vi "Parse Results (table).vi"(8 "error in (no error)":errorcluster, 11 "Instrument.Lockin":refnum<class "Instrument.Lockin.lvclass">) -> (0 "error out":errorcluster, 1 "Table":string[][](table), 2 "Results (Dictionary)":cluster{"key":string, "value":dbl}[](array[cluster]), 3 "Instrument.Lockin out":refnum<class "Instrument.Lockin.lvclass">)   [LabVIEW 2019, in "Instrument.Lockin.lvclass"]
uses:
  Instrument.Lockin.lvclass
  Typedefs/Results Type--Enum.ctl
  Instrument.Lockin.lvclass/Instrument.Lockin.ctl
  Instrument.DAQ/Typedefs/DAQ.Config.AI.Range--enum.ctl
  Instrument.DAQ/Instrument.DAQ.lvclass
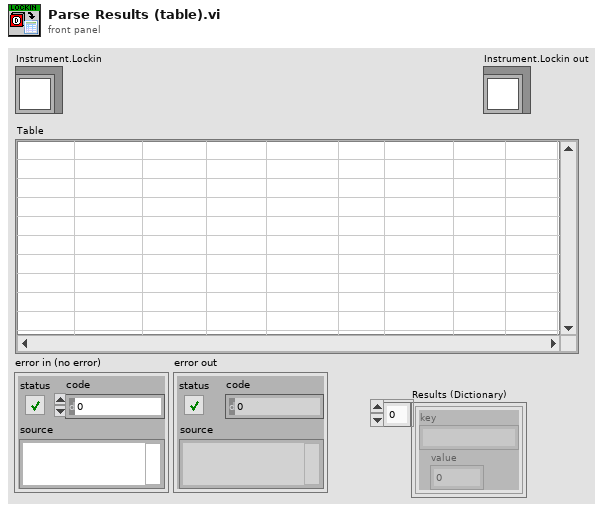
[diagram p1: front panel]
types:
  T1 = typedef "Instrument.Lockin.lvclass/Results Type--Enum.ctl" = enum16{"X", "Y", "R", "Theta", "Mean"}
  T2 = enum32{"Bad", "Idle", "Run top level", "Running"}
  T3 = typedef "Instrument.DAQ.lvclass/DAQ.Config.AI--Cluster--Array.ctl" = T4[]
  T4 = typedef "Instrument.DAQ.lvclass/DAQ.Config.AI--Cluster.ctl" = cluster{"Channels":tag, "Coupling":T5, "Range":T6, "input terminal configuration":i32, "Type":T7}
  T5 = typedef "Instrument.DAQ.lvclass/DAQ.Config.AI.Coupling--enum.ctl" = u16
  T6 = typedef "Instrument.DAQ.lvclass/DAQ.Config.AI.Range--enum.ctl" = enum16{"±0.316", "±1.00", "±3.16", "±10.0", "±31.6", "±42.4"}
  T7 = typedef "Instrument.DAQ.lvclass/DAQ.Type--enum.ctl" = enum16{"None", "USB 4431", "PXI 446x"}
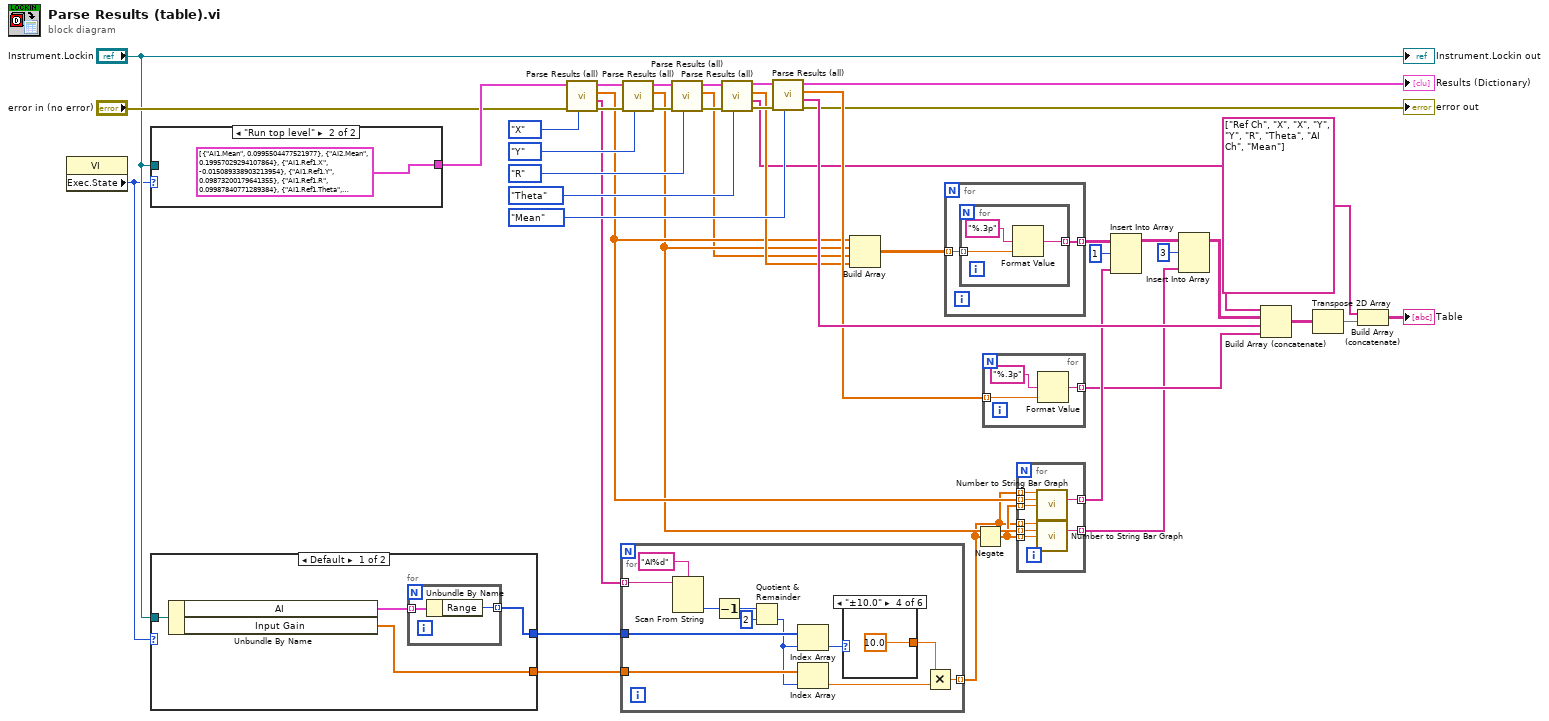
[diagram p0: block diagram]
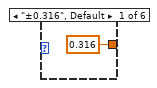
[diagram p2: hidden frame]
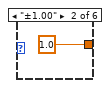
[diagram p3: hidden frame]
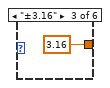
[diagram p4: hidden frame]
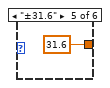
[diagram p5: hidden frame]
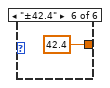
[diagram p6: hidden frame]
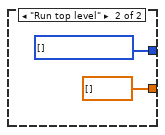
[diagram p7: hidden frame]
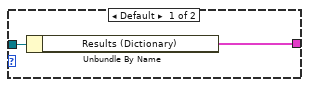
[diagram p8: hidden frame]
diagram:
  n1 = property class="VI"() -> ("Exec.State"=w3:T2)  [unwired: 2 in, 2 out]
  n2 = case shown="\"Run top level\"" w3 {
    tunnel: [w45 cluster{"key":string, "value":dbl}[] [{"key"="AI1.Mean", "value"=0.0995504477521977}, {"key"="AI2.Mean", "value"=0.19957029294107864}, {"key"="AI1.Ref1.X", "value"=-0.015089338903213954}, {"key"="AI1.Ref1.Y", "value"=0.09873200179641355}, {"key"="AI1.Ref1.R", "value"=0.09987840771289384}, {"key"="AI1.Ref1.Theta", "value"=98.68935048220581}, {"key"="AI2.Ref1.X", "value"=0.0007846947023169867}, {"key"="AI2.Ref1.Y", "value"=-0.0005938592767695586}, {"key"="AI2.Ref1.R", "value"=0.0009840805944888902}, {"key"="AI2.Ref1.Theta", "value"=-37.11854407465412}] ("Results.Results (Dictionary)")] -> w44
    tunnel: "Instrument.Lockin" -> [w46 _]
    frame Default {
      n3 = Unbundle By Name(w46) -> ("Results (Dictionary)"=w45:cluster{"key":string, "value":dbl}[])
    }
    frame "Run top level" {
    }
  }
  n4 = case shown="Default" w3 {
    tunnel: "Instrument.Lockin" -> [w51 _]
    tunnel: [w49 w55] -> w2
    tunnel: [w48 dbl[] [] ("Input Gain")] -> w1
    frame Default {
      n5 = Unbundle By Name(w51) -> ("AI"=w50:T3, "Input Gain"=w48:dbl[])
      n6 = for {
        tunnel: w50 -> [w53] mode=indexing
        tunnel: [w52] -> w49 mode=indexing
        n7 = Unbundle By Name(w53) -> ("Range"=w52:T6)
      }
    }
    frame "Run top level" {
      w55 = T6[] [] items=["±0.316", "±1.00", "±3.16", "±10.0", "±31.6", "±42.4"]
    }
  }
  n8 = call "Parse Results (all).vi"("Type"=Results_Type--Enum."X", "error in (no error)"="error in (no error)", "Results (Dictionary)"=w44) -> ("error out"=w43:errorcluster, "Names"=w11:string[], "Data"=w19:dbl[], "Results (Dictionary)"=w42:cluster{"key":string, "value":dbl}[])  [unwired: 5 in]
  n9 = for {
    tunnel: w11 -> [w67] mode=indexing
    tunnel: w2 -> [w62]
    tunnel: w1 -> [w61]
    tunnel: [w57] -> w9 mode=indexing
    n10 = Scan From String(format string="AI%d", input string=w67) -> (output 1=w65:i32)  [unwired: 3 in, 3 out]
    n11 = Decrement(x=w65) -> (x-1=w64:i32)
    n12 = Quotient & Remainder(x=w64, y=2) -> (floor(x/y)=w56:i32)  [unwired: 1 out]
    n13 = Index Array(array=w62, index=w56) -> (element=w60:T6)
    n14 = Index Array(array=w61, index=w56) -> (element=w58:dbl)
    n15 = case shown="\"±10.0\"" w60 {
      tunnel: [0.316 1.0 3.16 10.0 31.6 42.4] -> w59
      frame "±0.316", Default {
      }
      frame "±1.00" {
      }
      frame "±3.16" {
      }
      frame "±10.0" {
      }
      frame "±31.6" {
      }
      frame "±42.4" {
      }
    }
    n16 = Multiply(x=w59, y=w58) -> (x*y=w57:dbl)
  }
  n17 = call "Parse Results (all).vi"("Type"=Results_Type--Enum."Y", "error in (no error)"=w43, "Results (Dictionary)"=w42) -> ("error out"=w41:errorcluster, "Data"=w18:dbl[], "Results (Dictionary)"=w40:cluster{"key":string, "value":dbl}[])  [unwired: 5 in, 1 out]
  n18 = call "Parse Results (all).vi"("Type"=Results_Type--Enum."R", "error in (no error)"=w41, "Results (Dictionary)"=w40) -> ("error out"=w36:errorcluster, "Data"=w17:dbl[], "Results (Dictionary)"=w37:cluster{"key":string, "value":dbl}[])  [unwired: 5 in, 1 out]
  n19 = call "Parse Results (all).vi"("Type"=Results_Type--Enum."Theta", "error in (no error)"=w36, "Results (Dictionary)"=w37) -> ("error out"=w39:errorcluster, "Names"=w7:string[], "Data"=w21:dbl[], "Results (Dictionary)"=w38:cluster{"key":string, "value":dbl}[])  [unwired: 5 in]
  n20 = call "Parse Results (all).vi"("Type"=Results_Type--Enum."Mean", "error in (no error)"=w39, "Results (Dictionary)"=w38) -> ("error out"=→"error out":errorcluster, "Names"=w30:string[], "Data"=w24:dbl[], "Results (Dictionary)"=→"Results (Dictionary)":cluster{"key":string, "value":dbl}[])  [unwired: 5 in]
  n21 = Build Array(w19, w18, w17, w21) -> (w25:dbl[][])
  n22 = for {
    tunnel: [w74] -> w16 mode=indexing
    tunnel: w25 -> [w75] mode=indexing
    n23 = for {
      tunnel: [w78] -> w74 mode=indexing
      tunnel: w75 -> [w77] mode=indexing
      n24 = Format Value(format string="%.3p", value (0)=w77) -> (output string=w78:string)  [unwired: 1 in]
    }
  }
  n25 = Negate(x=w9) -> (-x=w10:dbl[])
  n26 = for {
    tunnel: w24 -> [w80] mode=indexing
    tunnel: [w79] -> w6 mode=indexing
    n27 = Format Value(format string="%.3p", value (0)=w80) -> (output string=w79:string)  [unwired: 1 in]
  }
  n28 = for {
    tunnel: w10 -> [w89] mode=indexing
    tunnel: w9 -> [w88] mode=indexing
    tunnel: w10 -> [w87] mode=indexing
    tunnel: w9 -> [w86] mode=indexing
    tunnel: w19 -> [w85] mode=indexing
    tunnel: w18 -> [w84] mode=indexing
    tunnel: [w83] -> w5 mode=indexing
    tunnel: [w82] -> w13 mode=indexing
    n29 = call "Number to String Bar Graph.vi"("Scale Max"=w86, "Numeric"=w85, "Scale Min"=w87) -> ("element"=w82:string)  [unwired: 12 in]
    n30 = call "Number to String Bar Graph.vi"("Scale Max"=w88, "Numeric"=w84, "Scale Min"=w89) -> ("element"=w83:string)  [unwired: 12 in]
  }
  n31 = Insert Into Array(array=w16, index (row)=1, new element=w13) -> (w14:string[][])  [unwired: 1 in]
  n32 = Insert Into Array(array=w14, index (row)=3, new element=w5) -> (w8:string[][])  [unwired: 1 in]
  n33 = Build Array (concatenate)(w7, w8, w30, w6) -> (w29:string[][])
  n34 = Transpose 2D Array(2D array=w29) -> (transposed array=w28:string[][])
  n35 = Build Array (concatenate)(string[] ["Ref Ch", "X", "X", "Y", "Y", "R", "Theta", "AI Ch", "Mean"] ("Names"), w28) -> (→"Table":string[][])
  "Instrument.Lockin out" <- "Instrument.Lockin"
